vi "Operate_JKISM_template_doc.vi"(6 "Save to md(F)/Load to vi(T)":bool=TRUE, 9 "Path":path=path "D:/github/JKI-State-Machine-Plus/src/help/NEVSTOP/JKI State Machine++/Template Description.md", 11 "vi path":path=path "D:/github/JKI-State-Machine-Plus/src/user.lib/_NEVSTOP/JKI State Machine++/JKISM++ No-Event Structure Template.vi") -> ()   [LabVIEW 2014]
panel:
  out "Array":cluster{refnum<vi>, "Text":string}[](array[cluster])
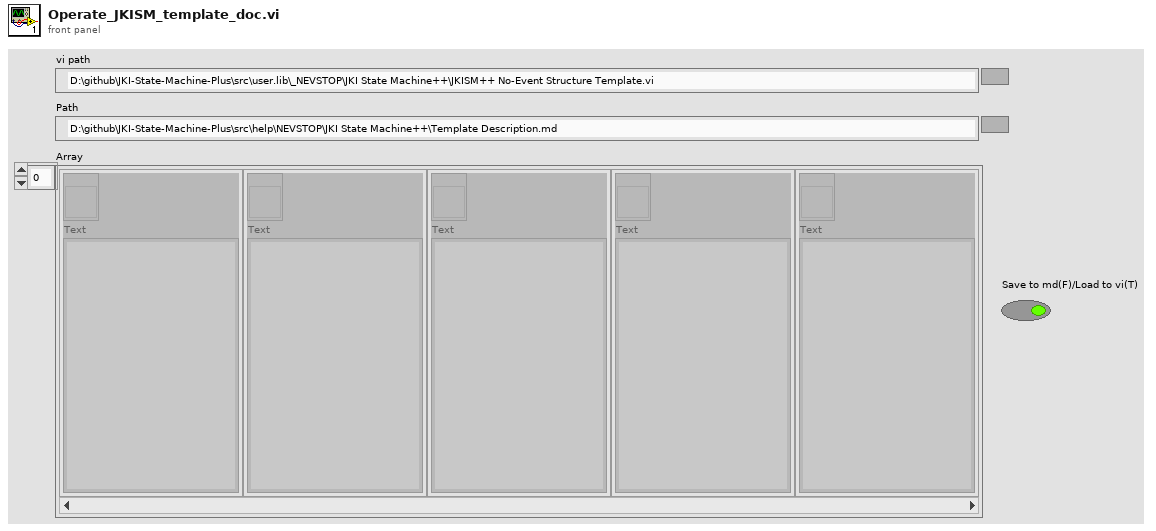
[diagram p1: front panel]
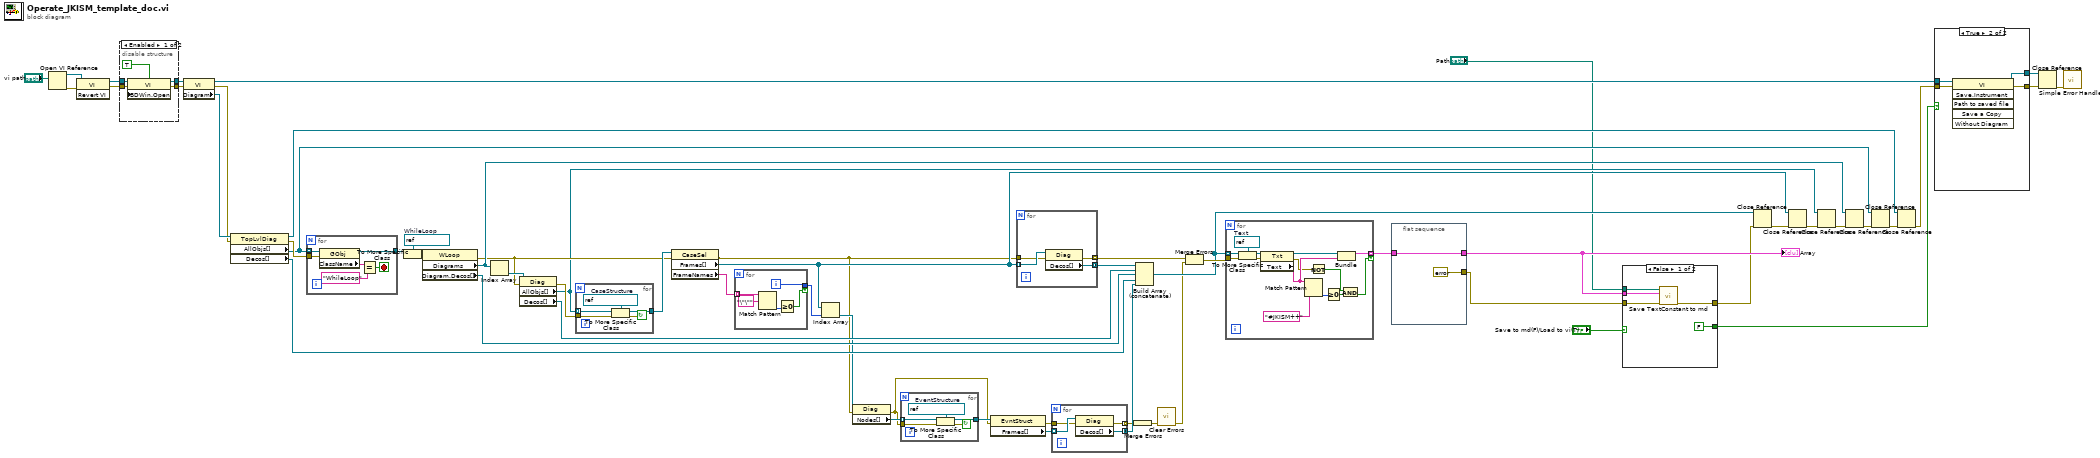
[diagram p0: block diagram]
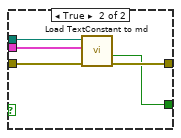
[diagram p3: hidden frame]
diagram:
  w50 = refnum<vi> refnum  # WhileLoop
  n1 = Open VI Reference(vi path="vi path") -> (vi reference=w59:refnum<vi>, error out=w60:errorcluster)  [unwired: 5 in]
  n2 = invoke class="VI" method="Revert VI"(reference=w59, error in=w60) -> (reference out=w42:refnum<vi>, error out=w41:errorcluster)  [unwired: 1 in, 1 out]
  n3 = disable-structure shown="Enabled" {
    disable-tunnel: w42 -> [w65 w67]
    disable-tunnel: w41 -> [w64 w66]
    disable-tunnel: [w63 w67] -> w40
    disable-tunnel: [w62 w66] -> w39
    frame Enabled {
      n4 = property class="VI"(reference=w65, error in=w64, "BDWin.Open"=TRUE ("Block Diagram Window:Open")) -> (reference out=w63:refnum<vi>, error out=w62:errorcluster)
    }
    frame Disabled {
    }
  }
  n5 = property class="VI"(reference=w40, error in=w39) -> (reference out=w58:refnum<vi>, error out=w53:errorcluster, "Diagram"=w54:refnum<vi>)
  n6 = property class="TopLvlDiag"(reference=w54, error in=w53) -> (reference out=w44:refnum<vi>, error out=w52:errorcluster, "AllObjs[]"=w46:refnum<vi>[], "Decos[]"=w20:refnum<vi>[])
  n7 = for {
    tunnel: w46 -> [w73] mode=indexing
    tunnel: w52 -> [w72]
    tunnel: [w71] -> w51
    stop <- w68 stop-if-true
    n8 = property class="GObj"(reference=w73, error in=w72) -> (reference out=w71:refnum<vi>, "ClassName"=w70:string)  [unwired: 1 out]
    n9 = Equal?(x=w70, y="WhileLoop") -> (x = y?=w68:bool)
  }
  n10 = To More Specific Class(target class=w50, reference=w51) -> (specific class reference=w49:refnum<vi>, error out=w48:errorcluster)  [unwired: 1 in]
  n11 = property class="WLoop"(reference=w49, error in=w48) -> (error out=w34:errorcluster, "Diagrams"=w38:refnum<vi>[], "Diagram.Decos[]"=w21:refnum<vi>[])  [unwired: 1 out]
  n12 = Index Array(array=w38) -> (element=w37:refnum<vi>)  [unwired: 1 in]
  n13 = property class="Diag"(reference=w37, error in=w34) -> (error out=w36:errorcluster, "AllObjs[]"=w30:refnum<vi>[], "Decos[]"=w23:refnum<vi>[])  [unwired: 1 out]
  n14 = for {
    tunnel: w30 -> [w78] mode=indexing
    tunnel: w36 -> [w77]
    tunnel: [w75] -> w35
    stop <- w76 continue-if-true
    w74 = refnum<vi> refnum  # CaseStructure
    n15 = To More Specific Class(target class=w74, reference=w78, error in=w77) -> (specific class reference=w75:refnum<vi>, error out=w76:errorcluster)
  }
  n16 = property class="CaseSel"(reference=w35, error in=w34) -> (error out=w9:errorcluster, "Frames[]"=w18:refnum<vi>[], "FrameNames"=w19:string[])  [unwired: 1 out]
  n17 = for {
    tunnel: w19 -> [w83] mode=indexing
    tunnel: [w81] -> w17 if=w79
    i -> [w81]
    n18 = Match Pattern(string=w83, regular expression="\"\"") -> (offset past match=w80:i32)  [unwired: 1 in, 3 out]
    n19 = Greater Or Equal To 0?(x=w80) -> (x >= 0?=w79:bool)
  }
  n20 = Index Array(array=w18, index=w17) -> (element=w16:refnum<vi>)
  n21 = property class="Diag"(reference=w16, error in=w9) -> (error out=w12:errorcluster, "Nodes[]"=w15:refnum<vi>[])  [unwired: 1 out]
  n22 = for {
    tunnel: w15 -> [w88] mode=indexing
    tunnel: w12 -> [w87]
    tunnel: [w85] -> w14
    stop <- w86 continue-if-true
    w84 = refnum<vi> refnum  # EventStructure
    n23 = To More Specific Class(target class=w84, reference=w88, error in=w87) -> (specific class reference=w85:refnum<vi>, error out=w86:errorcluster)
  }
  n24 = property class="EvntStruct"(reference=w14, error in=w12) -> (error out=w11:errorcluster, "Frames[]"=w13:refnum<vi>[])  [unwired: 1 out]
  n25 = for {
    tunnel: w18 -> [w92] mode=indexing
    tunnel: w9 -> [w91]
    tunnel: [w90] -> w27 mode=indexing
    tunnel: [w89] -> w24 mode=concatenating
    n26 = property class="Diag"(reference=w92, error in=w91) -> (error out=w90:errorcluster, "Decos[]"=w89:refnum<vi>[])  [unwired: 1 out]
  }
  n27 = for {
    tunnel: w13 -> [w96] mode=indexing
    tunnel: w11 -> [w95]
    tunnel: [w94] -> w8 mode=indexing
    tunnel: [w93] -> w10 mode=concatenating
    n28 = property class="Diag"(reference=w96, error in=w95) -> (error out=w94:errorcluster, "Decos[]"=w93:refnum<vi>[])  [unwired: 1 out]
  }
  n29 = Merge Errors(w8) -> (w7:errorcluster)
  n30 = Build Array (concatenate)(w24, w23, w21, w20, w10) -> (w22:refnum<vi>[])
  n31 = call <vilib>:"Clear Errors.vi"("error in (no error)"=w7) -> ("error out"=w6:errorcluster)  [unwired: 6 in]
  n32 = Merge Errors(w27, w6) -> (w25:errorcluster)
  n33 = for {
    tunnel: w22 -> [w110] mode=indexing
    tunnel: w25 -> [w109]
    tunnel: [w103] -> w26 mode=indexing if=w99
    w108 = refnum<vi> refnum  # Text
    n34 = To More Specific Class(target class=w108, reference=w110, error in=w109) -> (specific class reference=w107:refnum<vi>, error out=w105:errorcluster)
    n35 = property class="Txt"(reference=w107, error in=w105) -> (reference out=w106:refnum<vi>, error out=w98:errorcluster, "Text"=w102:string)
    n36 = Match Pattern(string=w102, regular expression="#JKISM++") -> (offset past match=w101:i32)  [unwired: 1 in, 3 out]
    n37 = Not(x=w98) -> (.not. x?=w97:bool)
    n38 = Greater Or Equal To 0?(x=w101) -> (x >= 0?=w100:bool)
    n39 = Bundle(w106, "Text"=w102) -> (w103:cluster{refnum<vi>, "Text":string})  [unwired: 1 in]
    n40 = And(x=w97, y=w100) -> (x .and. y?=w99:bool)
  }
  n41 = flat-sequence {
    tunnel: w26 -> [w111]
    tunnel: [errorcluster {"status"=FALSE, "code"=0, "source"=""} ("error in (no error)")] -> w4
    tunnel: [w111] -> w28
    frame #0 {
    }
  }
  n42 = case shown="False" "Save to md(F)/Load to vi(T)" {
    tunnel: w28 -> [w117 w121]
    tunnel: "Path" -> [w116 w120]
    tunnel: w4 -> [w115 w122]
    tunnel: [w114 w119] -> w3
    tunnel: [FALSE w118] -> w1
    frame False {
      n43 = call "Save TextConstant to md.vi"("error in (no error) 2"=w115, "Array 2"=w117, "Path 2"=w116) -> ("error out 2"=w114:errorcluster)  [unwired: 8 in]
    }
    frame True {
      n44 = call "Load TextConstant to md.vi"("error in (no error)"=w122, "Array"=w121, "Path"=w120) -> ("error out"=w119:errorcluster, "logical AND"=w118:bool)  [unwired: 7 in]
    }
  }
  n45 = Close Reference(reference=w22, error in (no error)=w3) -> (error out=w33:errorcluster)
  n46 = Close Reference(reference=w18, error in (no error)=w33) -> (error out=w32:errorcluster)
  n47 = Close Reference(reference=w30, error in (no error)=w32) -> (error out=w31:errorcluster)
  n48 = Close Reference(reference=w38, error in (no error)=w31) -> (error out=w47:errorcluster)
  n49 = Close Reference(reference=w46, error in (no error)=w47) -> (error out=w45:errorcluster)
  n50 = Close Reference(reference=w44, error in (no error)=w45) -> (error out=w43:errorcluster)
  n51 = case shown="True" w1 {
    tunnel: w58 -> [w123 w128]
    tunnel: [w124 w127] -> w57
    tunnel: [w123 w126] -> w56
    tunnel: w43 -> [w124 w125]
    frame False {
    }
    frame True {
      n52 = invoke class="VI" method="Save.Instrument"(reference=w128, error in=w125) -> (reference out=w126:refnum<vi>, error out=w127:errorcluster)  [unwired: 4 in, 4 out]
    }
  }
  n53 = Close Reference(reference=w56, error in (no error)=w57) -> (error out=w55:errorcluster)
  n54 = call <vilib>:"Simple Error Handler.vi"("error in (no error)"=w55) -> ()  [unwired: 4 in, 5 out]
  "Array" <- w28
